vi "MJTemplate.vi"(0 "VISA IN":refnum<visa-resource-name>, 5 "error in":errorcluster) -> (14 "VISA Out":refnum<visa-resource-name>, 19 "error out":errorcluster)   [LabVIEW 2018, in "PNA-X.lvlib"]
uses:
  PNA-X.lvlib
panel:
  in  "FileName":string
  in  "FileType":string(combo)="CSA"
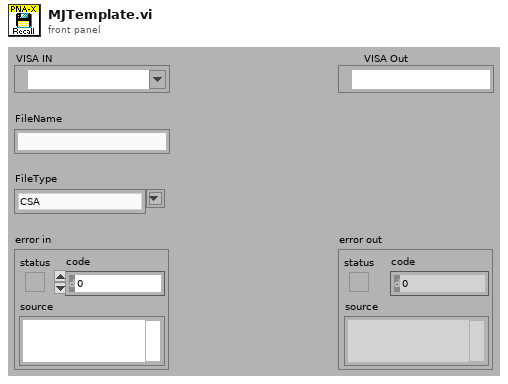
[diagram p1: front panel]
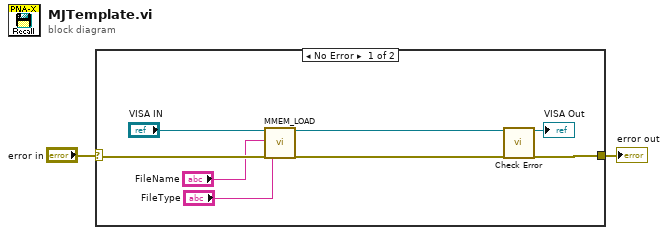
[diagram p0: block diagram]
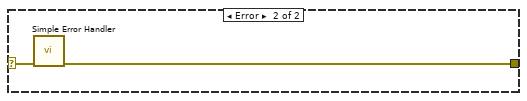
[diagram p2: hidden frame]
diagram:
  n1 = case shown="No Error" "error in" {
    selector: "error in" -> [w8 w12]
    tunnel: [w10 w11] -> w2
    frame No Error {
      n2 = call "MMEM_LOAD.vi"("VISA IN"="VISA IN", "FileName"="FileName", "error in"=w8, "FileType"="FileType") -> ("VISA Out"=w5:refnum<visa-resource-name>, "error out"=w7:errorcluster)  [unwired: 14 in]
      n3 = call "Check Error.vi"("VISA Resource Name"=w5, "error in (no error)"=w7) -> ("dup VISA session"=→"VISA Out":refnum<visa-resource-name>, "error out"=w10:errorcluster)  [unwired: 16 in]
    }
    frame Error {
      n4 = call <vilib>:"Simple Error Handler.vi"("error in (no error)"=w12) -> ("error out"=w11:errorcluster)  [unwired: 4 in, 4 out]
    }
  }
  "error out" <- w2
